vi "Get Project from Application Instance.vi"(8 "error in (no error)":errorcluster) -> (0 "error out":errorcluster, 2 "Open Projects":path[](array[path]))   [LabVIEW 2020, in "Execution UI.lvclass"]
uses:
  Execution UI.lvclass
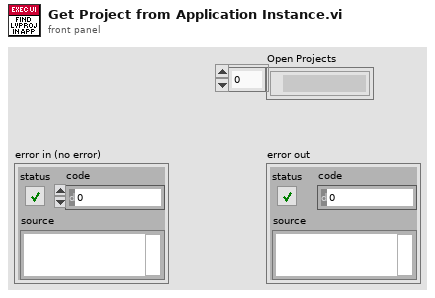
[diagram p1: front panel]
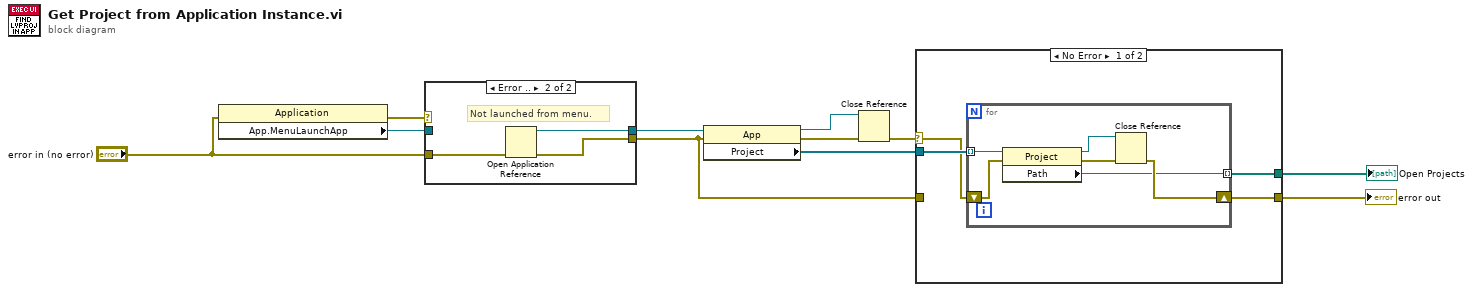
[diagram p0: block diagram]
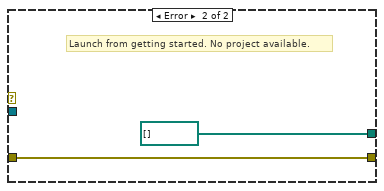
[diagram p2: hidden frame]
diagram:
  n1 = property class="Application"(error in="error in (no error)") -> (error out=w8:errorcluster, "App.MenuLaunchApp"=w7:refnum<vi>)  [unwired: 1 in, 1 out]
  n2 = case shown="Error .." w8 {
    selector: w8 -> [w12 _]
    tunnel: [w13 w16] -> w6
    tunnel: w7 -> [w13 _]
    tunnel: [w12 w15] -> w2
    tunnel: "error in (no error)" -> [_ w14]
    frame No Error {
      # "Launch from menu"
    }
    frame Error {
      # "Not launched from menu."
      n3 = Open Application Reference(8:w14) -> (0:w15:errorcluster, 3:w16:refnum<vi>)  [unwired: 3 in]
    }
  }
  n4 = property class="App"(reference=w6, error in=w2) -> (reference out=w11:refnum<vi>, error out=w10:errorcluster, "Project"=w9:refnum<vi>[])
  n5 = Close Reference(reference=w11, error in (no error)=w10) -> (error out=w5:errorcluster)
  n6 = case shown="No Error" w5 {
    selector: w5 -> [w19 _]
    tunnel: w9 -> [w20 _]
    tunnel: [w18 w28] -> w4
    tunnel: w2 -> [_ w28]
    tunnel: [w17 path[] [] ("Path")] -> w1
    frame No Error {
      n7 = for {
        tunnel: w20 -> [w24] mode=indexing
        shift-right: [w23] -> w18
        shift-left: w19 -> [w22]
        tunnel: [w21] -> w17 mode=indexing
        n8 = property class="Project"(reference=w24, error in=w22) -> (reference out=w26:refnum<vi>, error out=w25:errorcluster, "Path"=w21:path)
        n9 = Close Reference(reference=w26, error in (no error)=w25) -> (error out=w23:errorcluster)
      }
    }
    frame Error {
      # "Launch from getting started. No project available."
    }
  }
  "error out" <- w4
  "Open Projects" <- w1
